vi "Laser DataTrans.vi"(11 "Strin":string) -> (3 "Read":dbl)   [LabVIEW 2019]
uses:
  <vilib>/gmath/NI_Gmath.lvlib
panel:
  out "substring before match":string
  out "xi used":dbl[](array[numeric]) format="%_6g"
  out "(hi.lo)":u16
  # "-6.56"
  # "-16.50"
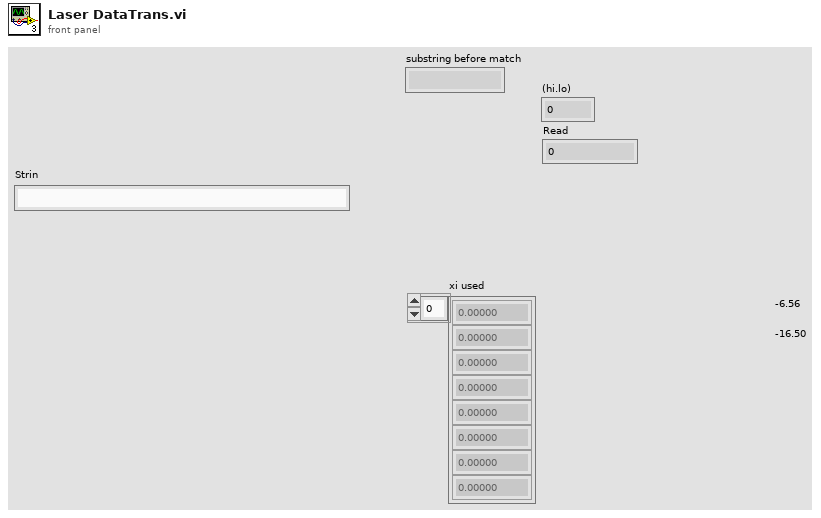
[diagram p1: front panel]
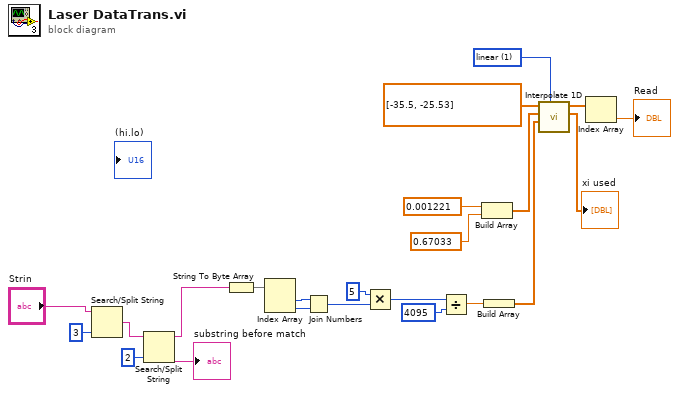
[diagram p0: block diagram]
diagram:
  w16 = 1 items=["nearest", "linear", "spline", "cubic Hermite", "Lagrange"] ("method")
  n1 = Search/Split String(string="Strin", offset (0)=3) -> (match + rest of string=w4:string)  [unwired: 1 in, 2 out]
  n2 = Search/Split String(string=w4, offset (0)=2) -> (substring before match=w2:string)  [unwired: 1 in, 2 out]
  "substring before match" <- w2
  n3 = String To Byte Array(string=w2) -> (unsigned byte array=w1:u8[])
  n4 = Index Array(array=w1) -> (element #1=w22:u8, element #2=w21:u8)  [unwired: 2 in]
  n5 = Join Numbers(hi=w22, lo=w21) -> ((hi.lo)=w20:u16)
  n6 = Multiply(x=u16 5, y=w20) -> (x*y=w18:u16)
  n7 = Divide(x=w18, y=u16 4095) -> (x/y=w7:dbl)
  n8 = Build Array(0.001221 ("x/y 3"), 0.67033 ("x/y 2")) -> (w13:dbl[])
  n9 = Build Array(w7) -> (w10:dbl[])
  n10 = call <vilib>:"Interpolate 1D.vi"("method"=w16, "xi"=w10, "X"=w13, "Y"=dbl[] [-35.5, -25.53]) -> ("xi used"=→"xi used":dbl[], "yi"=w9:dbl[])  [unwired: 5 in, 1 out]
  n11 = Index Array(array=w9) -> (element=→"Read":dbl)  [unwired: 1 in]
